vi "Initialize TreeBrowserWF.vi"(7 "Generate?":bool, 8 "error in (no error)":errorcluster, 9 "Input Channels":T1[](array[typedef]) {"Data Type" items=["Signed", "Unsigned", "IEEE Float"]}, 10 "Node Pointer":T2, 11 "TreeBrowserRef":refnum<k24>) -> (0 "error out":errorcluster, 2 "Channels":variant, 3 "TreeBrowserRef 2":refnum<k24>)   [LabVIEW 2021, in "LIN Frame Protection Addon System Explorer.lvlib"]
uses:
  LIN Frame Protection Addon System Explorer.lvlib
  <vilib>/NI VeriStand/Custom Device API/Custom Device Pointer.ctl
  NationalInstruments.VeriStand.SystemStorage
  Shared/Types/InputChannelConfiguration.ctl
  NationalInstruments.VeriStand.SystemStorageUI
  NationalInstruments.VeriStand
  <vilib>/NI VeriStand/Custom Device API/Custom Device API.lvlib
  Shared/LIN Frame Protection Addon Shared.lvlib
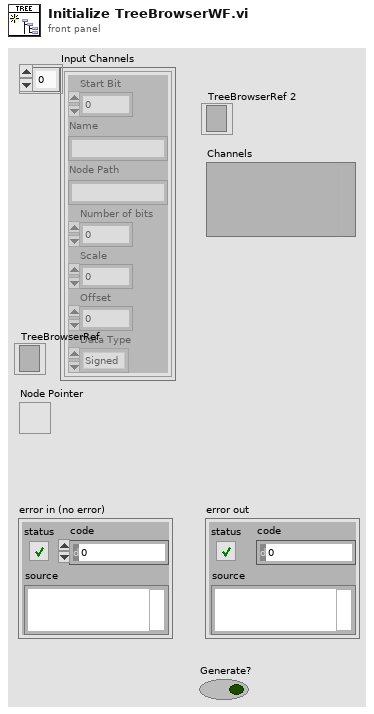
[diagram p1: front panel]
types:
  T1 = typedef "LIN Frame Protection Addon Shared.lvlib/InputChannelConfiguration.ctl" = cluster{"Start Bit":i32, "Name":string, "Node Path":string, "Number of bits":i32, "Scale":dbl, "Offset":dbl, "Data Type":u32}
  T2 = typedef "Custom Device API.lvlib/Custom Device Pointer.ctl" = refnum<k24>
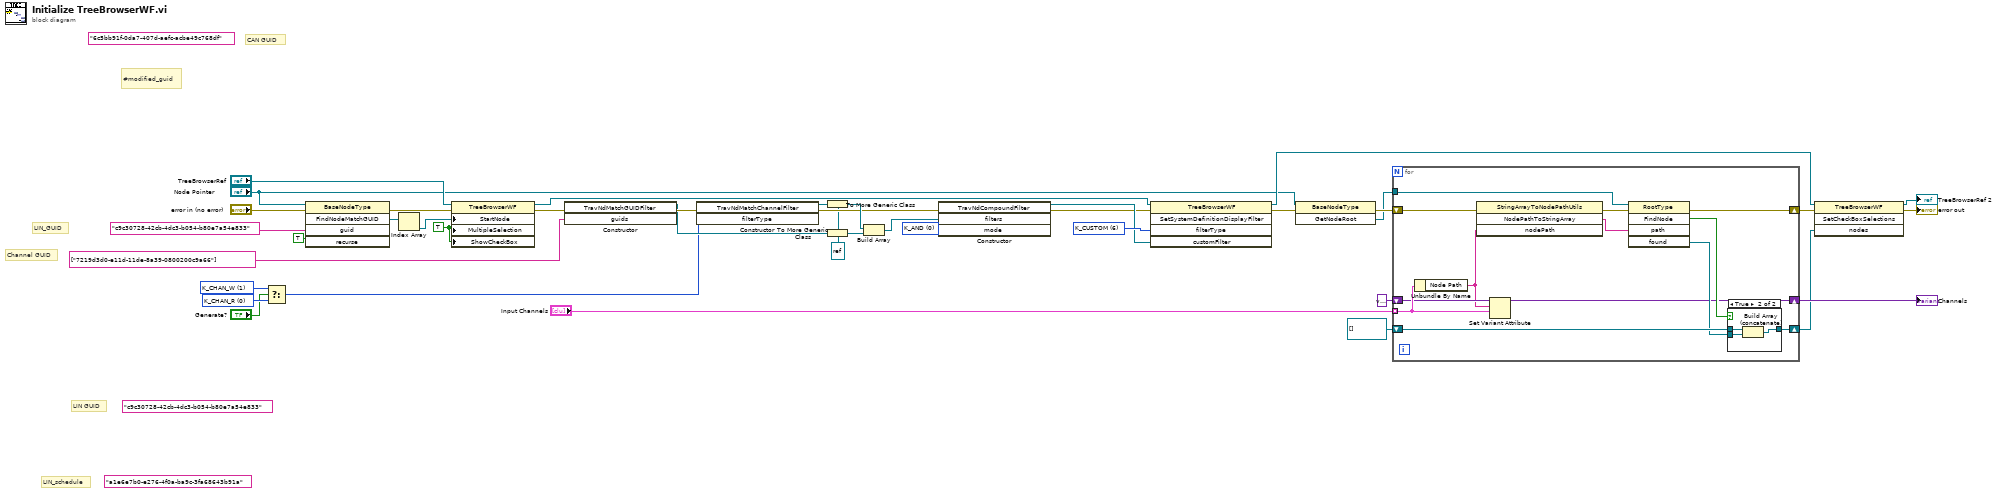
[diagram p0: block diagram]
diagram:
  (unwired) "a1e6e7b0-e276-4f0a-ba9c-3fa68643b91a" ("guid")
  (unwired) "c9c30728-42cb-4dc3-b054-b80e7a54e833" ("guid")
  (unwired) "6c5bb91f-0da7-407d-aefc-acbe49c768df" ("guid")
  w7 = refnum<k24> refnum
  w12 = 0 items=["K_AND", "K_OR"] ("mode")
  w15 = u8 0 items=["K_CHAN_R", "K_CHAN_W", "K_CHAN_VOLT", "K_CHAN_FAULT"] ("filterType")
  w16 = u8 1 items=["K_CHAN_R", "K_CHAN_W", "K_CHAN_VOLT", "K_CHAN_FAULT"] ("filterType")
  w34 = TRUE ("MultipleSelection")
  w25 = u8 6 items=["K_CHAN_R", "K_CHAN_W", "K_CHAN_RW", "K_CHAN_VOLT", "K_CHAN_FAULT", "K_ALL", "K_CUSTOM", "K_CHAN_R_VIS", "K_CHAN_W_VIS", "K_CHAN_RW_VIS", "K_CHAN_VOLT_VIS", "K_CHAN_FAULT_VIS", "K_WAVE", "K_WAVE_VIS", "K_WAVE_DBL", "K_WAVE_CDB", "K_WAVE_DBL_VIS", "K_WAVE_CDB_VIS"] ("filterType")
  # "LIN_schedule"
  # "LIN GUID"
  # "#modified_guid"
  # "Channel GUID"
  # "LIN_GUID"
  # "CAN GUID"
  n1 = Select(t=w16, s="Generate?", f=w15) -> (s? t:f=w1:u8)
  n2 = invoke class="BaseNodeType" method="FindNodeMatchGUID"(reference="Node Pointer", error in="error in (no error)", "guid"="c9c30728-42cb-4dc3-b054-b80e7a54e833", "recurse"=TRUE) -> (error out=w18:errorcluster, "FindNodeMatchGUID"=w21:refnum<k24>[])  [unwired: 1 in, 3 out]
  n3 = Index Array(array=w21) -> (element=w20:refnum<k24>)  [unwired: 1 in]
  n4 = property class="TreeBrowserWF"(reference="TreeBrowserRef", error in=w18, "StartNode"=w20, "MultipleSelection"=w34, "ShowCheckBox"=w34) -> (reference out=w27:refnum<k24>, error out=w24:errorcluster)
  n5 = constructor class="TravNdMatchGUIDFilter"(error in=w24, "guids"=string[] ["7219d3d0-e11d-11de-8a39-0800200c9a66"]) -> (reference out=w4:refnum<k24>, error out=w5:errorcluster)  [unwired: 2 in, 2 out]
  n6 = constructor class="TravNdMatchChannelFilter"(error in=w5, "filterType"=w1) -> (reference out=w6:refnum<k24>, error out=w8:errorcluster)  [unwired: 2 in, 2 out]
  n7 = To More Generic Class(target class=w7, reference=w6) -> (generic class reference=w10:refnum<k24>)
  n8 = To More Generic Class(target class=w7, reference=w4) -> (generic class reference=w11:refnum<k24>)
  n9 = Build Array(w10, w11) -> (w9:refnum<k24>[])
  n10 = constructor class="TravNdCompoundFilter"(error in=w8, "filters"=w9, "mode"=w12) -> (reference out=w3:refnum<k24>, error out=w2:errorcluster)  [unwired: 2 in, 3 out]
  n11 = invoke class="TreeBrowserWF" method="SetSystemDefinitionDisplayFilter"(reference=w27, error in=w2, "filterType"=w25, "customFilter"=w3) -> (reference out=w29:refnum<k24>, error out=w39:errorcluster)  [unwired: 1 in, 3 out]
  n12 = invoke class="BaseNodeType" method="GetNodeRoot"(reference="Node Pointer", error in=w39) -> (error out=w40:errorcluster, "GetNodeRoot"=w38:refnum<k24>)  [unwired: 1 in, 1 out]
  n13 = for {
    shift-right: [w50] -> w33
    shift-left: w40 -> [w42]
    tunnel: "Input Channels" -> [w45] mode=indexing
    tunnel: w38 -> [w53]
    shift-right: [w47] -> w35
    shift-left: refnum<k24>[] [] -> [w48]
    shift-right: [w43] -> w37
    shift-left: variant -> [w44]
    n14 = Unbundle By Name(w45) -> ("Node Path"=w41:string)
    n15 = invoke class="StringArrayToNodePathUtils" method="NodePathToStringArray"(error in=w42, "nodePath"=w41) -> (error out=w51:errorcluster, "NodePathToStringArray"=w52:string[])  [unwired: 2 in, 2 out]
    n16 = Set Variant Attribute(Variant=w44, name=w41, value=w45) -> (Variant out=w43:variant)  [unwired: 1 in, 2 out]
    n17 = invoke class="RootType" method="FindNode"(reference=w53, error in=w51, "path"=w52) -> (error out=w50:errorcluster, "FindNode"=w49:bool, "found"=w46:refnum<k24>)  [unwired: 2 in, 2 out]
    n18 = case shown="True" w49 {
      tunnel: w48 -> [w54 w57]
      tunnel: [w54 w55] -> w47
      tunnel: w46 -> [_ w56]
      frame False {
      }
      frame True {
        n19 = Build Array (concatenate)(w57, w56) -> (w55:refnum<k24>[])
      }
    }
  }
  "Channels" <- w37
  n20 = invoke class="TreeBrowserWF" method="SetCheckBoxSelections"(reference=w29, error in=w33, "nodes"=w35) -> (reference out=→"TreeBrowserRef 2":refnum<k24>, error out=→"error out":errorcluster)  [unwired: 1 in, 2 out]
